vi "Select Positions from ENUM.vi"(7 "PoseList":T1={"MotionMaster Ver"=0, "Pose List"=[{"Pose"=enum."None-Unknown", "Target"={"Lift"=0, "Extend"=0, "Wrist"=0}}, {"Pose"=enum."Intake", "Target"={"Lift"=326, "Extend"=-6481, "Wrist"=723}}, {"Pose"=enum."Score High", "Target"={"Lift"=970, "Extend"=-11200, "Wrist"=810}}, {"Pose"=enum."Score Mid", "Target"={"Lift"=910, "Extend"=-3500, "Wrist"=1417}}, {"Pose"=enum."Safe Position", "Target"={"Lift"=500, "Extend"=-500, "Wrist"=10}}, {"Pose"=enum."Home Pos", "Target"={"Lift"=154, "Extend"=-500, "Wrist"=10}}]}, 11 "Pose":T3) -> (3 "Selectet  Position Out":T4={"Lift"=154, "Extend"=-50, "Wrist"=10})   [LabVIEW 2020]
uses:
  ENUM_Pose List.ctl
  Shared Code/TypeDefs/Cluster_Pose Positions.ctl
  Shared Code/TypeDefs/Cluster_MotionMaster_Config Data.ctl
  Shared Code/TypeDefs/Cluster_Pose Name and  Data.ctl
  MotionMaster_SubCMD.lvlib
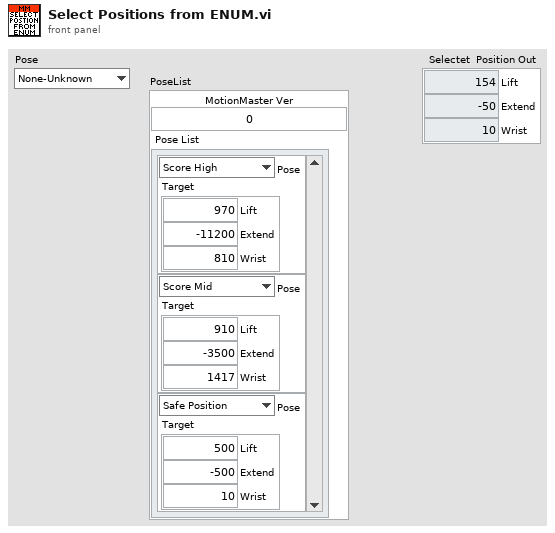
[diagram p1: front panel]
types:
  T1 = typedef "Cluster_MotionMaster_Config Data.ctl" = cluster{"MotionMaster Ver":u64, "Pose List":T2[]}
  T2 = typedef "Cluster_Pose Name and  Data.ctl" = cluster{"Pose":T3, "Target":T4}
  T3 = typedef "MotionMaster_SubCMD.lvlib/ENUM_Pose List.ctl" = enum16{"None-Unknown", "Intake", "Score High", "Score Mid", "Safe Position", "Home Pos"}
  T4 = typedef "Cluster_Pose Positions.ctl" = cluster{"Lift":i32, "Extend":i32, "Wrist":i32}
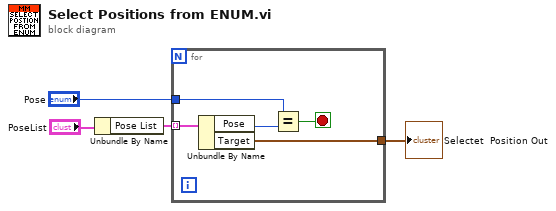
[diagram p0: block diagram]
diagram:
  n1 = Unbundle By Name("PoseList") -> ("Pose List"=w2:T2[])
  n2 = for {
    tunnel: "Pose" -> [w7]
    tunnel: w2 -> [w9] mode=indexing
    tunnel: [w5] -> w1
    stop <- w6 stop-if-true
    n3 = Unbundle By Name(w9) -> ("Pose"=w8:T3, "Target"=w5:T4)
    n4 = Equal?(x=w7, y=w8) -> (x = y?=w6:bool)
  }
  "Selectet  Position Out" <- w1
